vi "sendEventsFromTcpClient.vi"(8 "error in (no error)":errorcluster, 10 "timeout ms (1000)":i32=1000, 11 "connectionID":refnum<k5>) -> (0 "error out":errorcluster, 2 "eventsOut":string[](array[string]), 3 "connectionID":refnum<k5>)   [LabVIEW 2018]
doc: "Generate events as JSON packets and send them to TCP server."
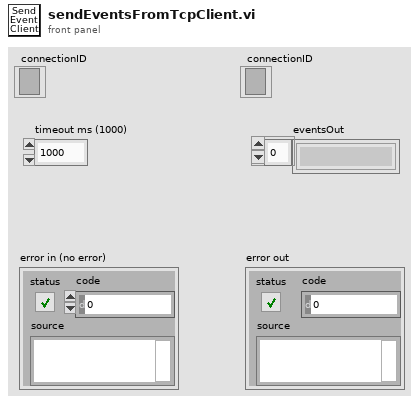
[diagram p1: front panel]
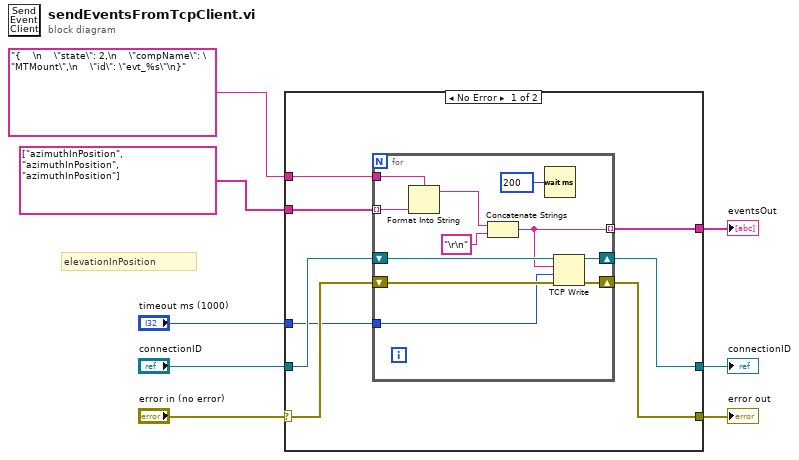
[diagram p0: block diagram]
diagram:
  # "elevationInPosition"
  n1 = case shown="No Error" "error in (no error)" {
    selector: "error in (no error)" -> [w11 w29]
    tunnel: [w14 w28] -> w8
    tunnel: [w13 w29] -> w6
    tunnel: "connectionID" -> [w16 w28]
    tunnel: "{    \n    \"state\": 2,\n    \"compName\": \"MTMount\",\n    \"id\": \"evt_%s\"\n}" ("Display") -> [w12 _]
    tunnel: string[] ["azimuthInPosition", "azimuthInPosition", "azimuthInPosition"] -> [w15 _]
    tunnel: [w10 _] -> w2
    tunnel: "timeout ms (1000)" -> [w9 _]
    frame No Error {
      n2 = for {
        shift-right: [w26] -> w13
        shift-left: w11 -> [w22]
        shift-right: [w24] -> w14
        shift-left: w16 -> [w23]
        tunnel: w12 -> [w21]
        tunnel: w15 -> [w20] mode=indexing
        tunnel: [w18] -> w10 mode=indexing
        tunnel: w9 -> [w17]
        n3 = Format Into String(format string=w21, w20) -> (resulting string=w19:string)  [unwired: 2 in, 1 out]
        n4 = Concatenate Strings(w19, "\r\n" ("string")) -> (w18:string)
        n5 = Wait (ms)(milliseconds to wait=u32 200) -> ()  [unwired: 1 out]
        n6 = TCP Write(connection ID=w23, data in=w18, error in (no error)=w22, 9:w17) -> (connection ID out=w24:refnum<k5>, error out=w26:errorcluster)  [unwired: 1 out]
      }
    }
    frame Error {
    }
  }
  "connectionID" <- w8
  "error out" <- w6
  "eventsOut" <- w2
